vi "Periodic Tasks.vi"(8 "error in":errorcluster) -> ()   [LabVIEW 2018]
doc: "This VI runs in parallel to other tasks. It can contain as many user-defined periodic loops as you need. These can carry out PID or other sorts of timed response."
uses:
  <vilib>/Rock Robotics/WPI/Solenoid/WPI_SolenoidValue.ctl
  RefNums_DriverStation.vi
  <vilib>/Rock Robotics/WPI/Utilities/WPI_GetSetVariantRefNum.vi
  Inputs_DriverStation.vi
  RefNums_Actuators.vi
  <vilib>/Rock Robotics/WPI/Solenoid/WPI_SolenoidSetEnum.vi
  <vilib>/Rock Robotics/WPI/RobotDrive/WPI_RobotDriveArcadeDrive_Standard(NoSaturation).vi
panel:
  out "BUTTERFLY":bool
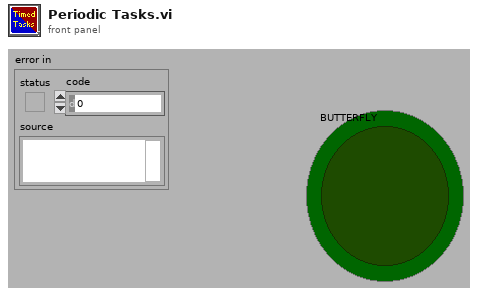
[diagram p1: front panel]
types:
  T1 = typedef "WPI_RobotDriveDevRef.ctl" = cluster{"DevStatus":errorcluster, "Motors[]":T2[], "Square Inputs":bool, "Max Output":dbl}
  T2 = typedef "WPI_MotorControlDeviceRef.ctl" = cluster{"DeviceStatus":errorcluster, "Type":T3, "PWM":cluster{"PWM Channel":T4, "DeadBand":T5}, "CAN":cluster{"Device Number":u8, "SetOutput VI Ref":variant, "GetOutput VI Ref":variant, "Enable VI Ref":variant, "Disable VI Ref":variant, "Data":variant}, "Invert":bool, "DIO PWM":cluster{"PWM \"Enable\" Channel":T4, "DIOChannel":T6, "PWM Rate":dbl}}
  T3 = typedef "WPI_MotorControlType.ctl" = enum16{"PWM", "CAN", "DIO PWM"}
  T4 = typedef "FPGA_DIOPWMChannel.ctl" = enum8{"PWM 0", "PWM 1", "PWM 2", "PWM 3", "PWM 4", "PWM 5", "PWM 6", "PWM 7", "PWM 8", "PWM 9", "PWM MXP 0", "PWM MXP 1", "PWM MXP 2", "PWM MXP 3", "PWM MXP 4", "PWM MXP 5", "PWM MXP 6", "PWM MXP 7", "PWM MXP 8", "PWM MXP 9", "Invalid"}
  T5 = typedef "WPI_PWMDeadband.ctl" = cluster{"Name":string, "maxPositivePwm":i32, "minPositivePwm":i32, "centerPwm":i32, "maxNegativePwm":i32, "minNegativePwm":i32, "angularRange":u16}
  T6 = typedef "FPGA_DIOChannel.ctl" = enum8{"DIO 0", "DIO 1", "DIO 2", "DIO 3", "DIO 4", "DIO 5", "DIO 6", "DIO 7", "DIO 8", "DIO 9", "DIO MXP 0", "DIO MXP 1", "DIO MXP 2", "DIO MXP 3", "DIO MXP 4", "DIO MXP 5", "DIO MXP 6", "DIO MXP 7", "DIO MXP 8", "DIO MXP 9", "DIO MXP 10", "DIO MXP 11", "DIO MXP 12", "DIO MXP 13", "DIO MXP 14", "DIO MXP 15", "SPI Port CS1", "SPI Port CS2", "SPI Port CS3", "SPI Port MISO", "SPI Port MOSI", "Invalid"}
  T7 = typedef "WPI_SolenoidDevRef.ctl" = cluster{"DevStatus":errorcluster, "Pneumatics Control Module":u8, "Forward Solenoid Channel":T8, "Reverse Solenoid Channel":T8}
  T8 = typedef "WPI_SolenoidChannel.ctl" = enum8{"Solenoid 0", "Solenoid 1", "Solenoid 2", "Solenoid 3", "Solenoid 4", "Solenoid 5", "Solenoid 6", "Solenoid 7", "Invalid"}
  T9 = typedef "WPI_JoystickDevRef.ctl" = cluster{"Device":T10}
  T10 = typedef "WPI_JoystickDeviceEnum.ctl" = enum16{"USB 0", "USB 1", "USB 2", "USB 3", "USB 4", "USB 5"}
  T11 = typedef "WPI_SolenoidValue.ctl" = enum16{"Off", "On", "Forward", "Reverse"}
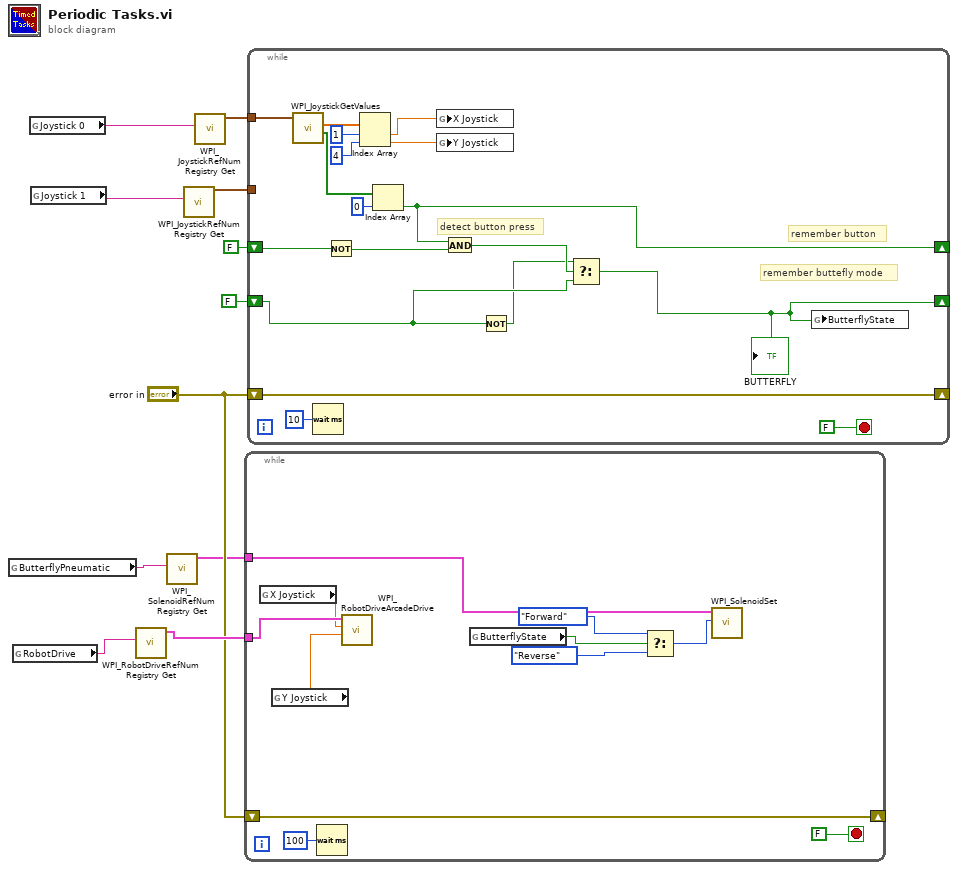
[diagram p0: block diagram]
diagram:
  n1 = global read "RefNums_Actuators.vi" "ButterflyPneumatic"() -> (w4:string)
  n2 = global read "RefNums_Actuators.vi" "RobotDrive"() -> (w7:string)
  n3 = global read "RefNums_DriverStation.vi" "Joystick 0"() -> (w10:string)
  n4 = global read "RefNums_DriverStation.vi" "Joystick 1"() -> (w8:string)
  n5 = call <vilib>:"WPI_RobotDriveRefNum Registry Get.vi"("refnum name"=w7) -> ("RobotDriveDevRef"=w6:T1)  [unwired: 9 in, 1 out]
  n6 = call <vilib>:"WPI_SolenoidRefNum Registry Get.vi"("refnum name"=w4) -> ("SolenoidDevRef"=w3:T7)  [unwired: 9 in, 1 out]
  n7 = call <vilib>:"WPI_JoystickRefNum Registry Get.vi"("refnum name"=w8) -> ("JoystickDevRef"=w9:T9)  [unwired: 9 in, 1 out]
  n8 = call <vilib>:"WPI_JoystickRefNum Registry Get.vi"("refnum name"=w10) -> ("JoystickDevRef"=w11:T9)  [unwired: 9 in, 1 out]
  n9 = while {
    tunnel: w6 -> [w20]
    shift-right: [w17] -> _
    shift-left: "error in" -> [w17]
    tunnel: w3 -> [w13]
    stop <- FALSE stop-if-true
    n10 = global read "Inputs_DriverStation.vi" "X Joystick"() -> (w19:dbl)
    n11 = global read "Inputs_DriverStation.vi" "Y Joystick"() -> (w18:dbl)
    n12 = Wait (ms)(milliseconds to wait=u32 100) -> ()  [unwired: 1 out]
    n13 = call-poly <vilib>:"WPI_RobotDriveArcadeDrive.vi"("Y axis value"=w18, "X axis value"=w19, "RobotDriveDevRef"=w20) -> ()  [unwired: 6 in, 3 out]
    n14 = global read "Inputs_DriverStation.vi" "ButterflyState"() -> (w12:bool)
    n15 = Select(t=WPI_SolenoidValue."Forward" ("Value"), s=w12, f=WPI_SolenoidValue."Reverse") -> (s? t:f=w14:T11)
    n16 = call-poly <vilib>:"WPI_SolenoidSet.vi"("Value"=w14, "SolenoidDevRef"=w13) -> ()  [unwired: 8 in, 2 out]
  }
  n17 = while {
    tunnel: w11 -> [w38]
    tunnel: w9 -> [_]
    shift-right: [w32] -> _
    shift-left: "error in" -> [w32]
    shift-right: [w29] -> _
    shift-left: FALSE -> [w28]
    shift-right: [w25] -> _
    shift-left: FALSE -> [w24]
    stop <- FALSE stop-if-true
    # "detect button press"
    # "remember buttefly mode"
    # "remember button"
    n18 = call <vilib>:"WPI_JoystickGetValues.vi"("JoystickDevRef"=w38) -> ("Buttons"=w31:bool[], "Axes"=w37:dbl[])  [unwired: 6 in, 3 out]
    n19 = Wait (ms)(milliseconds to wait=u32 10) -> ()  [unwired: 1 out]
    n20 = Not(x=w28) -> (.not. x?=w27:bool)
    n21 = Index Array(array=w37, index #1=1 ("index"), index #2=4 ("index")) -> (element #1=w34:dbl, element #2=w33:dbl)
    n22 = Index Array(array=w31, index=0) -> (element=w29:bool)
    n23 = global write "Inputs_DriverStation.vi" "X Joystick"(w34) -> ()
    n24 = global write "Inputs_DriverStation.vi" "Y Joystick"(w33) -> ()
    n25 = And(x=w29, y=w27) -> (x .and. y?=w26:bool)
    n26 = Not(x=w24) -> (.not. x?=w23:bool)
    n27 = Select(t=w23, s=w26, f=w24) -> (s? t:f=w25:bool)
    "BUTTERFLY" <- w25
    n28 = global write "Inputs_DriverStation.vi" "ButterflyState"(w25) -> ()
  }
